vi "gatherPelvicVars.vi"() -> (0 "BoundaryYpelv":dbl[](array[numeric]), 1 "BoundaryXPelv":dbl[](array[numeric]), 2 "pel_cn":dbl[](array[numeric]), 3 "viconData_2":dbl[](array[numeric]), 4 "K constant_pel":dbl, 8 "FM --- FF_pel":dbl[](array[numeric]))   [LabVIEW 2017]
panel:
  out "BoundaryZpelv":dbl[](array[numeric])
  # "Pelvis Variables for 3D FF"
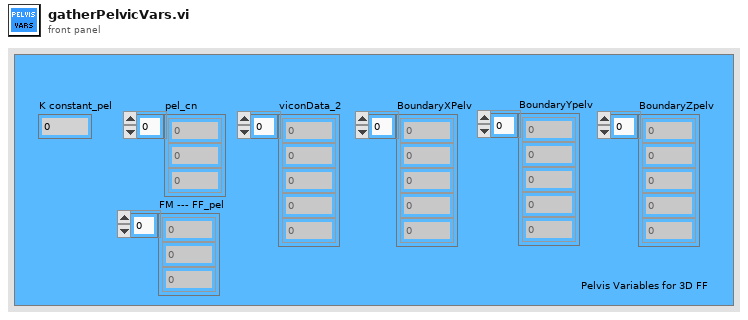
[diagram p1: front panel]
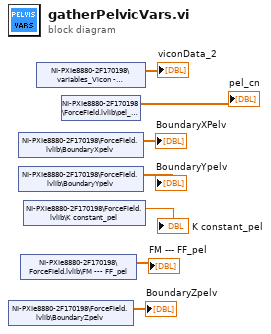
[diagram p0: block diagram]
diagram:
  n1 = shared-variable "NI-PXIe8880-2F170198\\ForceField.lvlib\\BoundaryZpelv"() -> (→"BoundaryZpelv":dbl[])  [unwired: 1 in, 1 out]
  n2 = shared-variable "NI-PXIe8880-2F170198\\ForceField.lvlib\\BoundaryXpelv"() -> (→"BoundaryXPelv":dbl[])  [unwired: 1 in, 1 out]
  n3 = shared-variable "NI-PXIe8880-2F170198\\ForceField.lvlib\\BoundaryYpelv"() -> (→"BoundaryYpelv":dbl[])  [unwired: 1 in, 1 out]
  n4 = shared-variable "NI-PXIe8880-2F170198\\ForceField.lvlib\\FM --- FF_pel"() -> (→"FM --- FF_pel":dbl[])  [unwired: 1 in, 1 out]
  n5 = shared-variable "NI-PXIe8880-2F170198\\ForceField.lvlib\\K constant_pel"() -> (→"K constant_pel":dbl)  [unwired: 1 in, 1 out]
  n6 = shared-variable "NI-PXIe8880-2F170198\\variables_Vicon - networkPublished.lvlib\\viconData_2"() -> (→"viconData_2":dbl[])  [unwired: 1 in, 1 out]
  n7 = shared-variable "NI-PXIe8880-2F170198\\ForceField.lvlib\\pel_cn"() -> (→"pel_cn":dbl[])  [unwired: 1 in, 1 out]
